vi "test Update Discrete Bit Field by Index.vi"(8 "error in (no error)":errorcluster, 11 "TestCase in":refnum<class "Discrete.lvclass">) -> (0 "error out":errorcluster, 3 "TestCase out":refnum<class "Discrete.lvclass">)   [LabVIEW 2027, in "Discrete.lvclass"]
uses:
  Discrete.lvclass
  6e1d2ac8-71cc-41db-b083-493d6063b283.vi
  6e1d2ac8-71cc-41db-b083-493d6063b283.vi/9935dc85-f143-411c-b80b-16b6c96eb14a.vi
  6e1d2ac8-71cc-41db-b083-493d6063b283.vi/b24d9be9-5807-4d59-88b8-dc532f996cb3.vi
  6e1d2ac8-71cc-41db-b083-493d6063b283.vi/e4a2156f-f189-4bbd-8a3a-9da1a7e591f8.vi
  C:/Program Files/National Instruments/LabVIEW 2027/vi.lib/addons/_JKI Toolkits/VI Tester/TestCase.llb/TestCase.lvclass
  <vilib>/addons/_JKI Toolkits/VI Tester/TestCase.llb/TestCase.lvclass
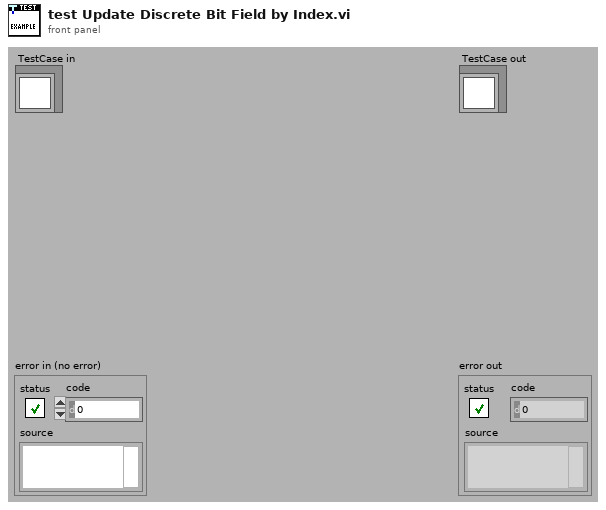
[diagram p1: front panel]
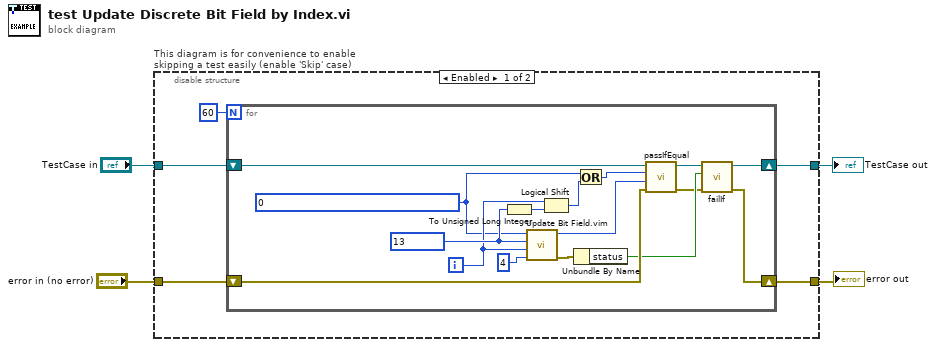
[diagram p0: block diagram]
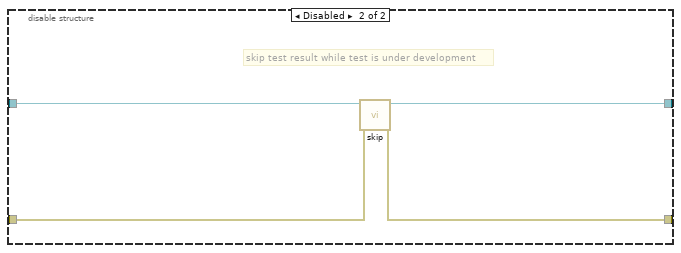
[diagram p2: hidden frame]
diagram:
  n1 = disable-structure "This diagram is for convenience to enable skipping a test easily (enable 'Skip' case)" shown="Enabled" {
    disable-tunnel: "TestCase in" -> [w9 w29]
    disable-tunnel: [w6 w27] -> w1
    disable-tunnel: [w7 w28] -> w3
    disable-tunnel: "error in (no error)" -> [w8 w26]
    frame Enabled {
      n2 = for {
        N: 60 -> [_]
        shift-right: [w14] -> w6
        shift-left: w9 -> [w25]
        shift-right: [w15] -> w7
        shift-left: w8 -> [w20]
        i -> [w13]
        w10 = u32 0 ("word in")
        w23 = u8 13 ("value")
        n3 = To Unsigned Long Integer(number=w23) -> (unsigned 32bit integer=w12:u32)
        n4 = call "Update Bit Field.vim"("bit field size"=4, "bit field start index"=w13, "value"=w23, "word in"=w10) -> ("error out"=w19:errorcluster, "word out"=w21:u32)  [unwired: 6 in]
        n5 = Logical Shift(y=w13, x=w12) -> (x << y=w11:u32)
        n6 = Unbundle By Name(w19) -> ("status"=w18:bool)
        n7 = Or(x=w10, y=w11) -> (x .or. y?=w22:u32)
        n8 = call-dynamic "passIfEqual.vi"("error in (no error)"=w20, "y"=w21, "x"=w22, "TestCase in"=w25) -> ("error out"=w16:errorcluster, "TestCase out"=w17:refnum<class "Discrete.lvclass">)  [unwired: 6 in]
        n9 = call-dynamic "failIf.vi"("error in (no error)"=w16, "fail"=w18, "TestCase in"=w17) -> ("error out"=w15:errorcluster, "TestCase out"=w14:refnum<class "Discrete.lvclass">)  [unwired: 7 in]
      }
    }
    frame Disabled {
      # "skip test result while test is under development"
      n10 = call <vilib>:"skip.vi"("error in (no error)"=w26, "TestCase in"=w29) -> ("error out"=w28:errorcluster, "TestCase out"=w27:refnum<class "Discrete.lvclass">)  [unwired: 8 in]
    }
  }
  "error out" <- w3
  "TestCase out" <- w1
